vi "Process Build VI Operation.vi"(6 "Caller VI Path":path, 7 "Assert Scripting Configuration":T1, 8 "error in (no error)":errorcluster, 10 "Discard?":bool) -> (0 "error out":errorcluster, 3 "Assert VI Path":path, 5 "Valid Configuration":bool)   [LabVIEW 2016]
uses:
  Assert Scripting Configuration.ctl
  <vilib>/Utility/Data Type/Type Definitions/Data Type.ctl
  <vilib>/Utility/Data Type/NI_Data Type.lvlib
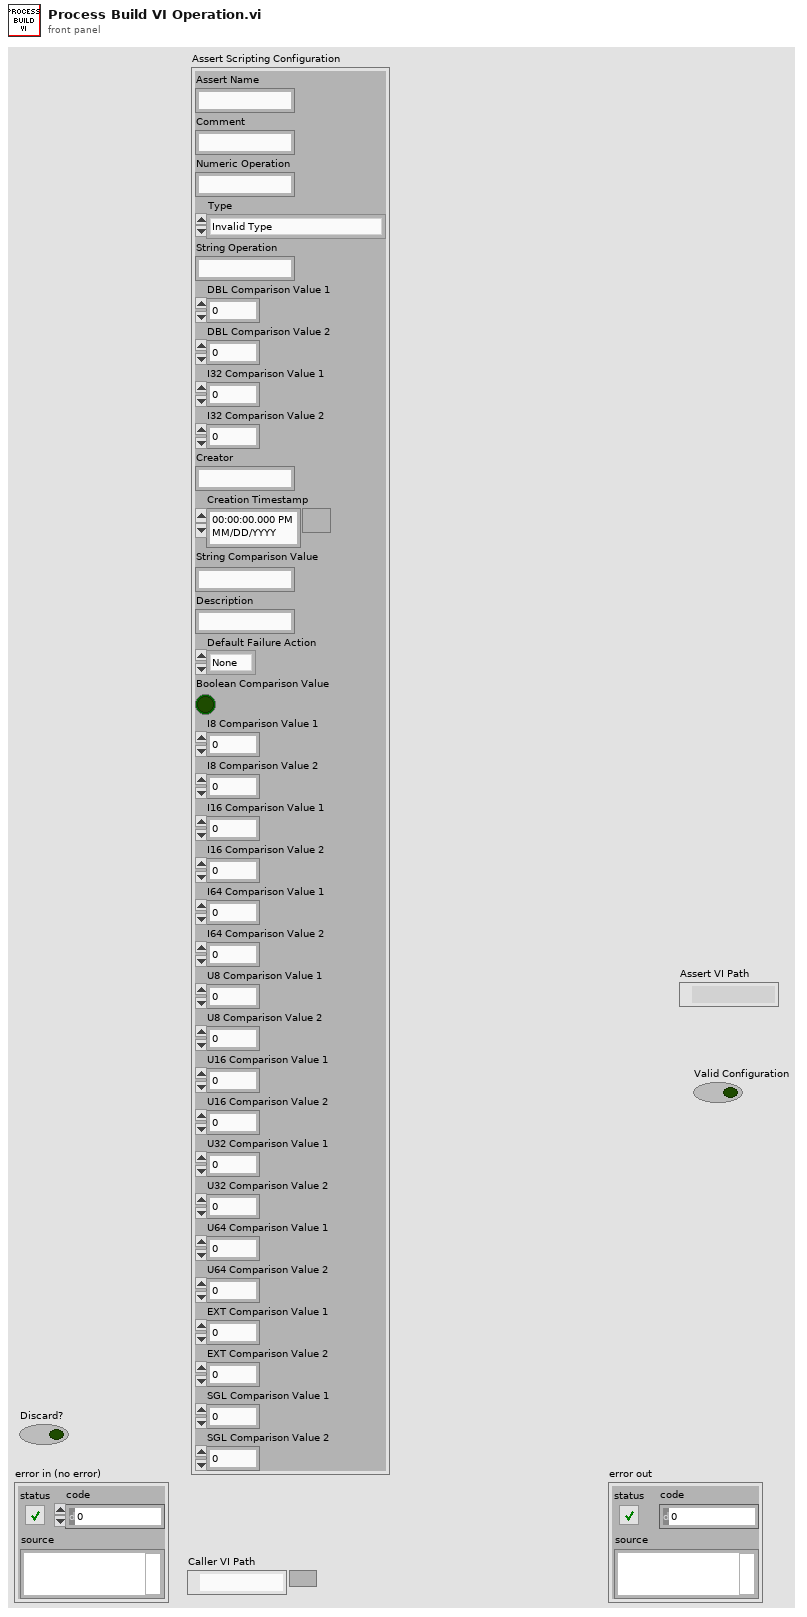
[diagram p1: front panel]
types:
  T1 = typedef "Assert Scripting Configuration.ctl" = cluster{"Assert Name":string, "Comment":string, "Numeric Operation":string, "Type":T2, "String Operation":string, "DBL Comparison Value 1":dbl, "DBL Comparison Value 2":dbl, "I32 Comparison Value 1":i32, "I32 Comparison Value 2":i32, "Creator":string, "Creation Timestamp":timestamp, "String Comparison Value":string, "Description":string, "Default Failure Action":enum16{"None", "Log To File", "Pause Execution", "Abort Execution"}, "Boolean Comparison Value":bool, "I8 Comparison Value 1":i8, "I8 Comparison Value 2":i8, "I16 Comparison Value 1":i16, "I16 Comparison Value 2":i16, "I64 Comparison Value 1":i64, "I64 Comparison Value 2":i64, "U8 Comparison Value 1":u8, "U8 Comparison Value 2":u8, "U16 Comparison Value 1":u16, "U16 Comparison Value 2":u16, "U32 Comparison Value 1":u32, "U32 Comparison Value 2":u32, "U64 Comparison Value 1":u64, "U64 Comparison Value 2":u64, "EXT Comparison Value 1":ext, "EXT Comparison Value 2":ext, "SGL Comparison Value 1":sgl, "SGL Comparison Value 2":sgl}
  T2 = typedef "NI_Data Type.lvlib/Data Type.ctl" = enum8{"Invalid Type", "Void", "I8", "I16", "I32", "I64", "U8", "U16", "U32", "U64", "Single Float", "Double Float", "Extended Float", "Single Complex", "Double Complex", "Extended Complex", "Enum U8", "Enum U16", "Enum U32", "Enum U64", "Single Float With Unit", "Double Float With Unit", "Extended Float With Unit", "Single Complex with Unit", "Double Complex with Unit", "Extended Complex with Unit", "Boolean", "String", "Path", "Picture", "Tag", "Array", "Cluster", "Variant", "LV Variant", "Waveform", "Timestamp", "Digital Waveform", "Digital Data", "ExpressData", "Refnum", "External Data", "VI", "Poly VI", "LabVIEW Class Instance", "Fixed Point"}
  T3 = enum16{"None", "Log To File", "Pause Execution", "Abort Execution"}
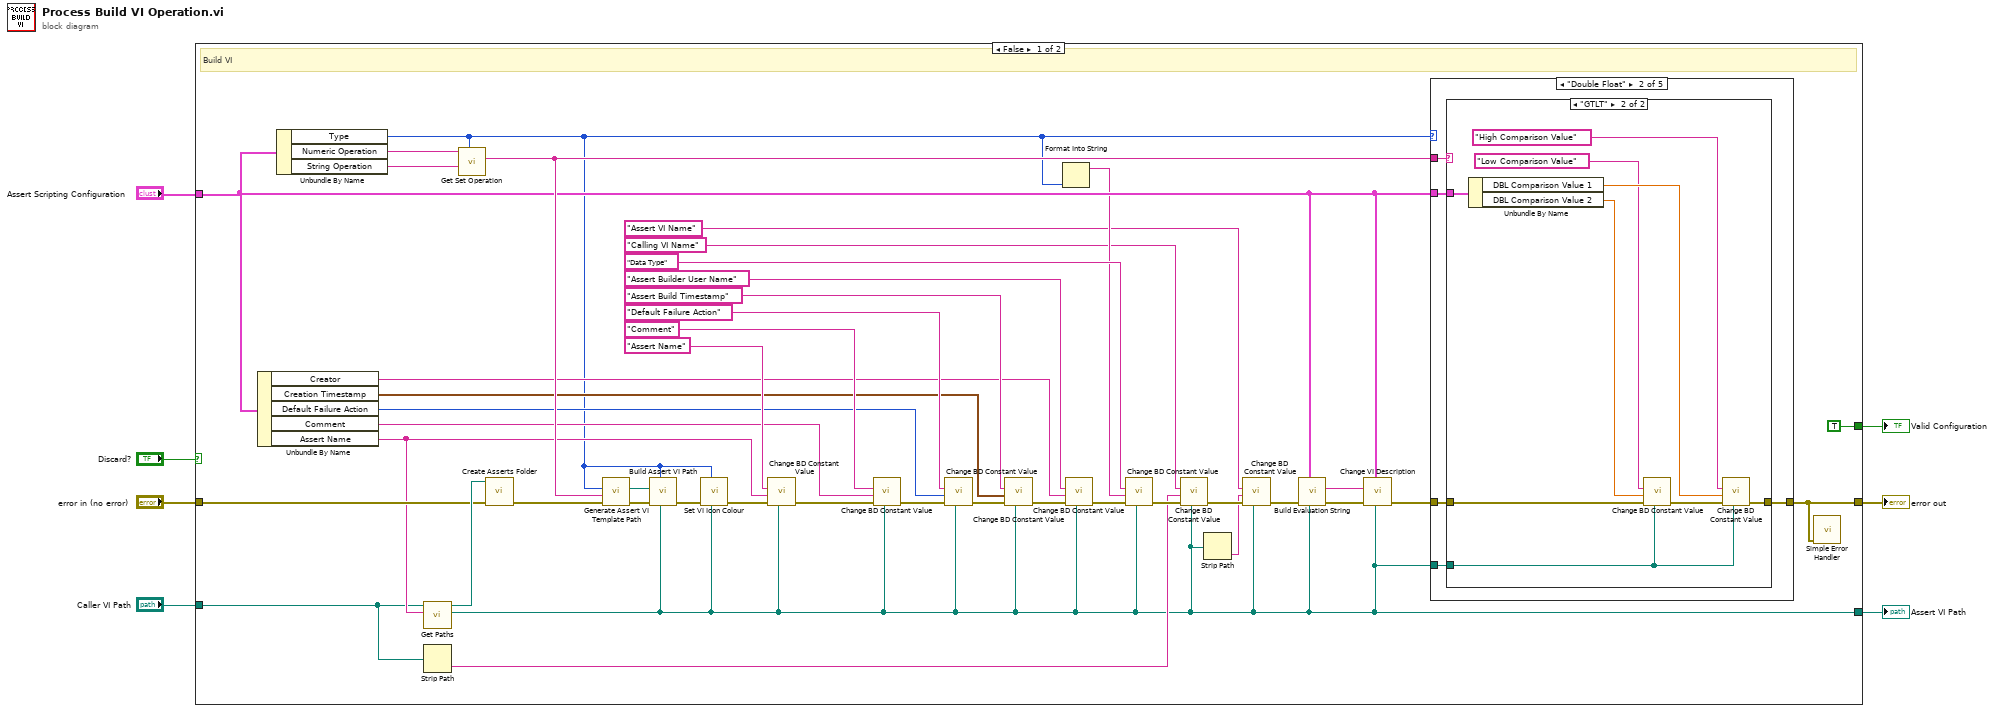
[diagram p0: block diagram]
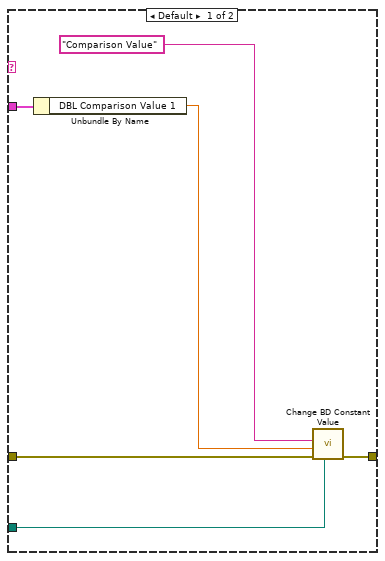
[diagram p3: hidden frame]
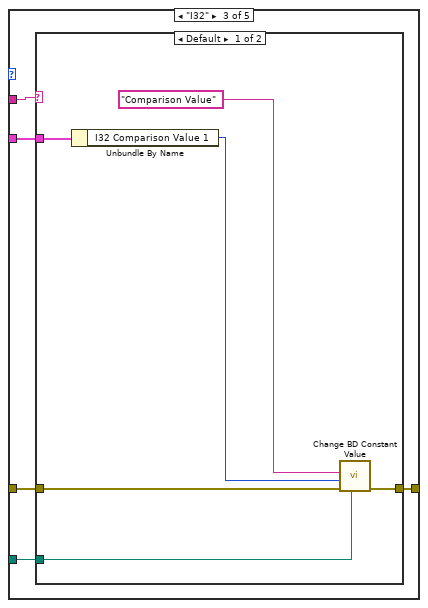
[diagram p4: hidden frame]
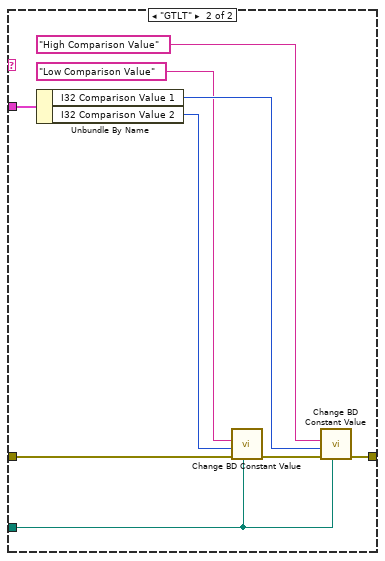
[diagram p5: hidden frame]
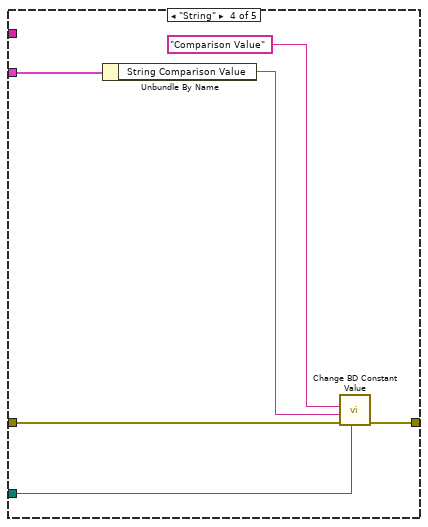
[diagram p6: hidden frame]
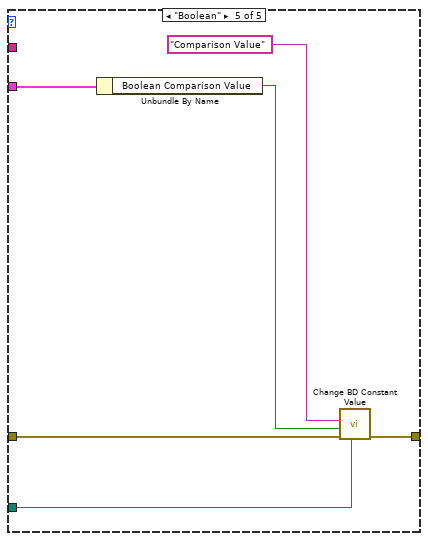
[diagram p7: hidden frame]
diagram:
  n1 = case shown="False" "Discard?" {
    tunnel: "error in (no error)" -> [w42 w104]
    tunnel: "Caller VI Path" -> [w12 _]
    tunnel: [w27 w104] -> w4
    tunnel: [w8 _] -> w5
    tunnel: [TRUE _] -> w6
    tunnel: "Assert Scripting Configuration" -> [w29 _]
    frame False {
      # "Build VI"
      n2 = Unbundle By Name(w29) -> ("Creator"=w18:string, "Creation Timestamp"=w19:timestamp, "Default Failure Action"=w31:T3, "Comment"=w35:string, "Assert Name"=w36:string)
      n3 = Unbundle By Name(w29) -> ("Type"=w9:T2, "Numeric Operation"=w39:string, "String Operation"=w38:string)
      n4 = call "Get Paths.vi"("Assert Name"=w36, "Path"=w12) -> ("Assert VI Path"=w8:path, "Asserts Folder Path"=w49:path)  [unwired: 8 in]
      n5 = Strip Path(path=w12) -> (name=w11:string)  [unwired: 1 out]
      n6 = call "Get Set Operation.vi"("Type"=w9, "String Operation"=w38, "Numeric Operation"=w39) -> ("Operation"=w37:string)  [unwired: 8 in]
      n7 = call "Create Asserts Folder.vi"("error in (no error)"=w42, "Folder Path"=w49) -> ("error out"=w43:errorcluster)  [unwired: 9 in]
      n8 = call "Generate Assert VI Template Path.vi"("error in (no error)"=w43, "Operation"=w37, "Data Type"=w9) -> ("error out"=w41:errorcluster, "Template Path"=w40:path)  [unwired: 7 in]
      n9 = call "Build Assert VI Path.vi"("Assert VI path"=w8, "Type"=w9, "error in (no error)"=w41, "Template Path"=w40) -> ("error out"=w50:errorcluster)  [unwired: 7 in]
      n10 = call "Set VI Icon Colour.vi"("VI Path"=w8, "Type"=w9, "error in (no error)"=w50) -> ("error out"=w10:errorcluster)  [unwired: 8 in]
      n11 = call "Change BD Constant Value.vi"("Assert VI Path"=w8, "error in (no error)"=w10, "Data Value"=w36, "Constant Name"="Assert Name") -> ("error out"=w45:errorcluster)  [unwired: 7 in]
      n12 = call "Change BD Constant Value.vi"("Assert VI Path"=w8, "error in (no error)"=w45, "Data Value"=w35, "Constant Name"="Comment") -> ("error out"=w44:errorcluster)  [unwired: 7 in]
      n13 = call "Change BD Constant Value.vi"("Assert VI Path"=w8, "error in (no error)"=w44, "Data Value"=w31, "Constant Name"="Default Failure Action") -> ("error out"=w33:errorcluster)  [unwired: 7 in]
      n14 = call "Change BD Constant Value.vi"("Assert VI Path"=w8, "error in (no error)"=w33, "Data Value"=w19, "Constant Name"="Assert Build Timestamp") -> ("error out"=w25:errorcluster)  [unwired: 7 in]
      n15 = Format Into String(w9) -> (resulting string=w20:string)  [unwired: 3 in, 1 out]
      n16 = call "Change BD Constant Value.vi"("Assert VI Path"=w8, "error in (no error)"=w25, "Data Value"=w18, "Constant Name"="Assert Builder User Name") -> ("error out"=w26:errorcluster)  [unwired: 7 in]
      n17 = call "Change BD Constant Value.vi"("Assert VI Path"=w8, "error in (no error)"=w26, "Data Value"=w20, "Constant Name"="Data Type") -> ("error out"=w24:errorcluster)  [unwired: 7 in]
      n18 = call "Change BD Constant Value.vi"("Assert VI Path"=w8, "error in (no error)"=w24, "Data Value"=w11, "Constant Name"="Calling VI Name") -> ("error out"=w17:errorcluster)  [unwired: 7 in]
      n19 = Strip Path(path=w8) -> (name=w13:string)  [unwired: 1 out]
      n20 = call "Change BD Constant Value.vi"("Assert VI Path"=w8, "error in (no error)"=w17, "Data Value"=w13, "Constant Name"="Assert VI Name") -> ("error out"=w16:errorcluster)  [unwired: 7 in]
      n21 = call "Build Evaluation String.vi"("VI Path"=w8, "Assert Scripting Configuration"=w29, "error in (no error)"=w16) -> ("error out"=w30:errorcluster, "Evaluation String"=w28:string)  [unwired: 7 in]
      n22 = call "Change VI Description.vi"("VI Path"=w8, "Assert Scripting Configuration"=w29, "error in (no error)"=w30, "Evaluation String"=w28) -> ("error out"=w34:errorcluster)  [unwired: 7 in]
      n23 = case shown="\"Double Float\"" w9 {
        tunnel: w8 -> [_ w54 w76 w93 w99]
        tunnel: w34 -> [w51 w55 w75 w97 w103]
        tunnel: [w51 w56 w74 w96 w102] -> w27
        tunnel: w29 -> [_ w53 w73 w95 w101]
        tunnel: w37 -> [_ w52 w72 _ _]
        frame Default {
        }
        frame "Double Float" {
          n24 = case shown="\"GTLT\"" w52 {
            tunnel: w54 -> [w57 w63]
            tunnel: w55 -> [w62 w71]
            tunnel: [w61 w67] -> w56
            tunnel: w53 -> [w60 w69]
            frame Default {
              n25 = Unbundle By Name(w60) -> ("DBL Comparison Value 1"=w59:dbl)
              n26 = call "Change BD Constant Value.vi"("Assert VI Path"=w57, "error in (no error)"=w62, "Data Value"=w59, "Constant Name"="Comparison Value") -> ("error out"=w61:errorcluster)  [unwired: 7 in]
            }
            frame "GTLT" {
              n27 = Unbundle By Name(w69) -> ("DBL Comparison Value 1"=w66:dbl, "DBL Comparison Value 2"=w68:dbl)
              n28 = call "Change BD Constant Value.vi"("Assert VI Path"=w63, "error in (no error)"=w71, "Data Value"=w68, "Constant Name"="Low Comparison Value") -> ("error out"=w70:errorcluster)  [unwired: 7 in]
              n29 = call "Change BD Constant Value.vi"("Assert VI Path"=w63, "error in (no error)"=w70, "Data Value"=w66, "Constant Name"="High Comparison Value") -> ("error out"=w67:errorcluster)  [unwired: 7 in]
            }
          }
        }
        frame "I32" {
          n30 = case shown="Default" w72 {
            tunnel: w76 -> [w77 w83]
            tunnel: w75 -> [w82 w91]
            tunnel: [w81 w87] -> w74
            tunnel: w73 -> [w80 w89]
            frame Default {
              n31 = Unbundle By Name(w80) -> ("I32 Comparison Value 1"=w79:i32)
              n32 = call "Change BD Constant Value.vi"("Assert VI Path"=w77, "error in (no error)"=w82, "Data Value"=w79, "Constant Name"="Comparison Value") -> ("error out"=w81:errorcluster)  [unwired: 7 in]
            }
            frame "GTLT" {
              n33 = Unbundle By Name(w89) -> ("I32 Comparison Value 1"=w86:i32, "I32 Comparison Value 2"=w88:i32)
              n34 = call "Change BD Constant Value.vi"("Assert VI Path"=w83, "error in (no error)"=w91, "Data Value"=w88, "Constant Name"="Low Comparison Value") -> ("error out"=w90:errorcluster)  [unwired: 7 in]
              n35 = call "Change BD Constant Value.vi"("Assert VI Path"=w83, "error in (no error)"=w90, "Data Value"=w86, "Constant Name"="High Comparison Value") -> ("error out"=w87:errorcluster)  [unwired: 7 in]
            }
          }
        }
        frame "String" {
          n36 = Unbundle By Name(w95) -> ("String Comparison Value"=w94:string)
          n37 = call "Change BD Constant Value.vi"("Assert VI Path"=w93, "error in (no error)"=w97, "Data Value"=w94, "Constant Name"="Comparison Value") -> ("error out"=w96:errorcluster)  [unwired: 7 in]
        }
        frame "Boolean" {
          n38 = Unbundle By Name(w101) -> ("Boolean Comparison Value"=w100:bool)
          n39 = call "Change BD Constant Value.vi"("Assert VI Path"=w99, "error in (no error)"=w103, "Data Value"=w100, "Constant Name"="Comparison Value") -> ("error out"=w102:errorcluster)  [unwired: 7 in]
        }
      }
      n40 = call <vilib>:"Simple Error Handler.vi"("error in (no error)"=w27) -> ()  [unwired: 4 in, 5 out]
    }
    frame True {
      # "Cancelled"
    }
  }
  "Valid Configuration" <- w6
  "Assert VI Path" <- w5
  "error out" <- w4
